vi "ExSubSetupCascadeADC.vi"(0 "Camera Handle":u32, 1 "Fast ADC":bool, 2 "ReadOut Port":u32 max=1 step=1, 3 "Avalanche Gain\nOnly valid for \nport 0":dbl format="%.2f", 4 "ADC Gain":u32, 5 "error in (no error)":errorcluster) -> (6 "Camera Handle":u32, 7 "ADC Speed (Khz)":u32, 8 "error out":errorcluster)   [LabVIEW 2010]
panel:
  # "Setup Cascade ADC\nThis sub VI sets the\nreadout port, Avlanche\ngain, ADC (fast or slow)\nand the gain for ADC.\nIt returns the ADC speed\nselected in Khz"
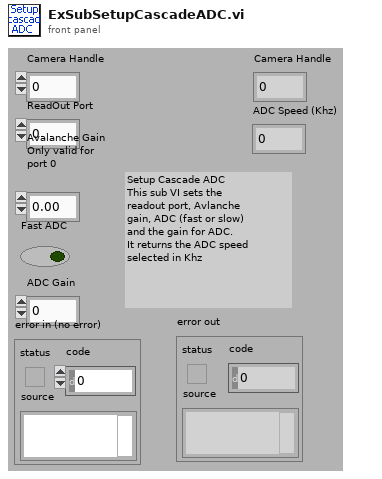
[diagram p1: front panel]
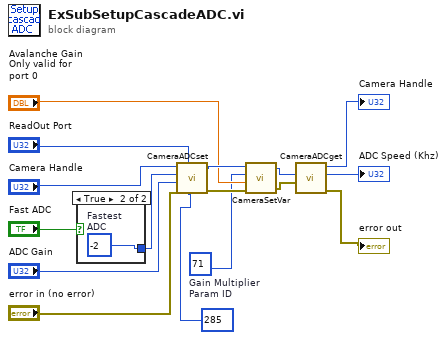
[diagram p0: block diagram]
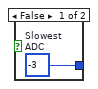
[diagram p2: hidden frame]
diagram:
  w7 = 71  # Gain Multiplier Param ID
  n1 = case shown="True" "Fast ADC" {
    tunnel: [w17 w18] -> w12
    frame False {
      w17 = -3  # Slowest ADC
    }
    frame True {
      w18 = -2  # Fastest ADC
    }
  }
  n2 = call <userlib>:"CameraADCset.vi"("ADC offset"=285, "Read Out port"="ReadOut Port", "error in (no error)"="error in (no error)", "ADC Gain"="ADC Gain", "ADC Speed"=w12, "Camera Handle"="Camera Handle") -> ("error out"=w10:errorcluster, "Camera Handle"=w9:u32)
  n3 = call <userlib>:"CameraSetVar.vi"("error in"=w10, "Value"="Avalanche Gain\nOnly valid for \nport 0", "Parameter ID"=w7, "Camera Handle"=w9) -> ("error out"=w6:errorcluster, "CameraHandle"=w5:u32)
  n4 = call <userlib>:"CameraADCget.vi"("Camera handle"=w5, "error in (no error)"=w6) -> ("Camera handle"=→"Camera Handle":u32, "ADC Speed"=→"ADC Speed (Khz)":i32, "error out"=→"error out":errorcluster)  [unwired: 5 out]
